vi "Start LabVIEW.vi"(8 "Error In":errorcluster, 11 "Install LV Data":T1={"SSH Session"=refnum, "Status Log"="", "Detailed Log"="", "Credentials"={"Hostname or IP"="192.168.7.2", "Username"="root", "Password"=""}, "Target Info"={"OS Version"="", "CPU"="", "Systemd Version"="", "Internet Access"=FALSE, "Device Type"="", "LV Installed Ver"="", "LV Available Ver"="", "LV Upgrade Available"=FALSE, "Hostname"="", "NIC Info"=[]}, "Reboot Required?"=FALSE}) -> (0 "Error Out":errorcluster, 1 "Log":string, 2 "LV Running?":bool, 3 "Install LV Data":T1={"SSH Session"=refnum, "Status Log"="", "Detailed Log"="", "Credentials"={"Hostname or IP"="192.168.7.2", "Username"="root", "Password"=""}, "Target Info"={"OS Version"="", "CPU"="", "Systemd Version"="", "Internet Access"=FALSE, "Device Type"="", "LV Installed Ver"="", "LV Available Ver"="", "LV Upgrade Available"=FALSE, "Hostname"="", "NIC Info"=[]}, "Reboot Required?"=FALSE})   [LabVIEW 2019, in "LMH-LINX.lvlib"]
uses:
  <vilib>/MakerHub/LINX/LMH-LINX.lvlib
  <vilib>/MakerHub/LINX/Private/Utilties/Target Management/Install LV Data.ctl
  E:/lv2019/dist/vi.lib/MakerHub/LINX/Resources/Renci.SshNet.dll
  Resources/Renci.SshNet.dll
  <vilib>/MakerHub/LINX/Private/Utilties/Target Management/Target Info.ctl
  <vilib>/MakerHub/LINX/Private/Utilties/Target Management/NIC Info.ctl
  <vilib>/MakerHub/LINX/Private/Utilties/Target Management/NIC Mode.ctl
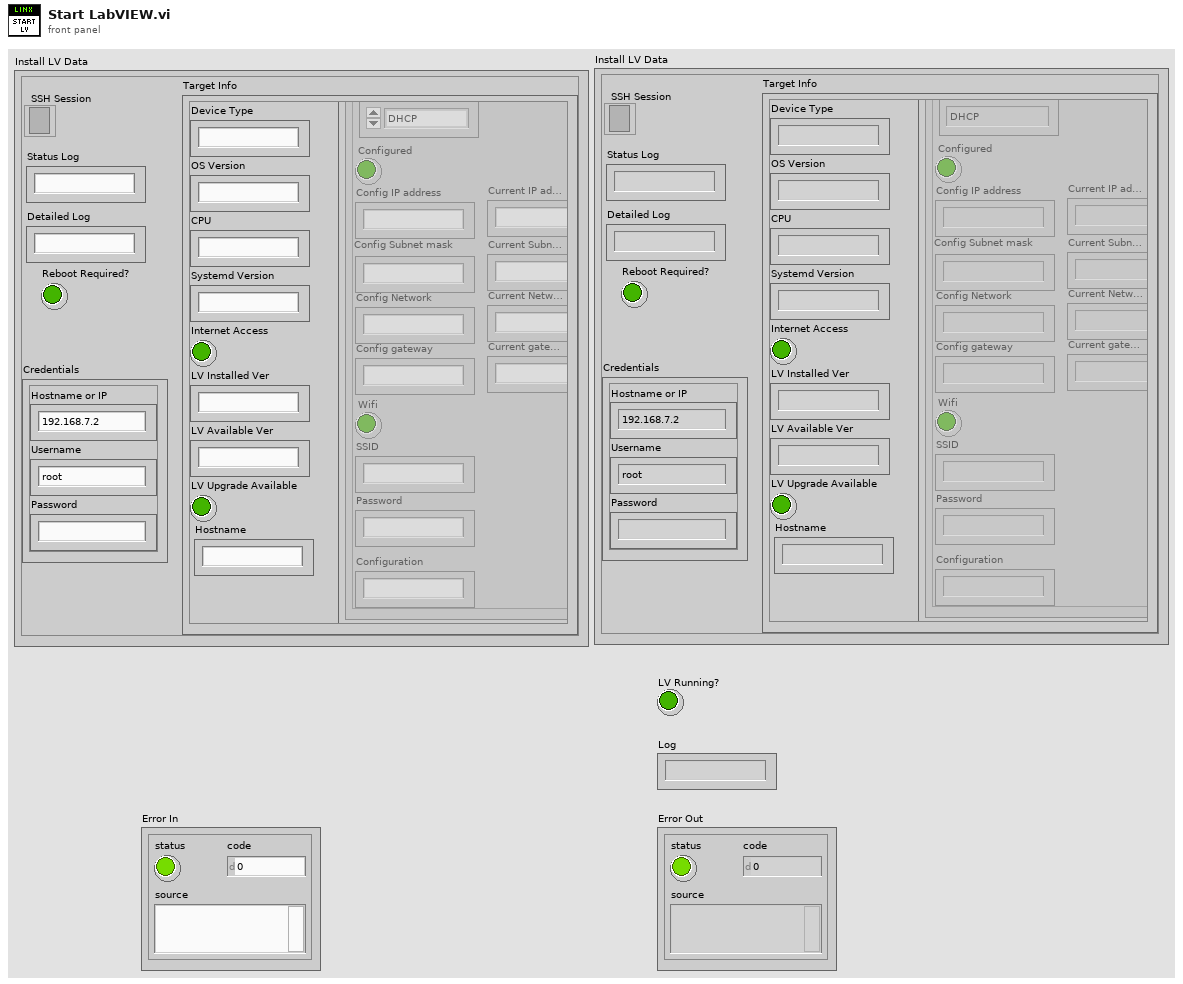
[diagram p1: front panel]
types:
  T1 = typedef "LMH-LINX.lvlib/Install LV Data.ctl" = cluster{"SSH Session":refnum<k24>, "Status Log":string, "Detailed Log":string, "Credentials":cluster{"Hostname or IP":string, "Username":string, "Password":string}, "Target Info":T2, "Reboot Required?":bool}
  T2 = typedef "LMH-LINX.lvlib/Target Info.ctl" = cluster{"OS Version":string, "CPU":string, "Systemd Version":string, "Internet Access":bool, "Device Type":string, "LV Installed Ver":string, "LV Available Ver":string, "LV Upgrade Available":bool, "Hostname":string, "NIC Info":T3[]}
  T3 = typedef "LMH-LINX.lvlib/NIC Info.ctl" = cluster{"Name":string, "NIC Mode":T4, "Configured":bool, "Config IP address":string, "Config Subnet mask":string, "Config Network":string, "Config gateway":string, "Wifi":bool, "SSID":string, "Password":string, "Configuration":string, "Current IP address":string, "Current Subnet mask":string, "Current gateway":string, "Current Network":string}
  T4 = typedef "LMH-LINX.lvlib/NIC Mode.ctl" = enum16{"DHCP", "Static", "Loopback"}
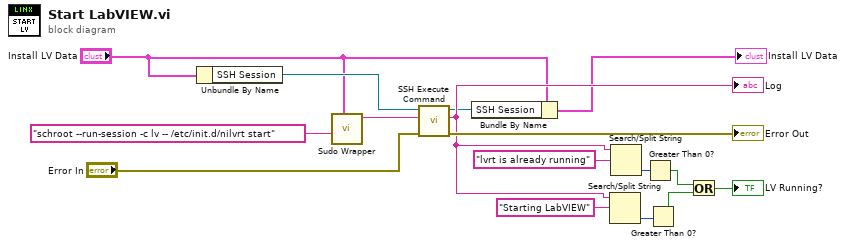
[diagram p0: block diagram]
diagram:
  n1 = Unbundle By Name("Install LV Data") -> ("SSH Session"=w6:refnum<k24>)
  n2 = call <vilib>:"Sudo Wrapper.vi"("Install LV Data"="Install LV Data", "comand string"="schroot --run-session -c lv -- /etc/init.d/nilvrt start") -> ("combined command string"=w2:string)  [unwired: 9 in]
  n3 = call <vilib>:"SSH Execute Command.vi"("Error In"="Error In", "Command"=w2, "SSH Session"=w6) -> ("Error Out"=→"Error Out":errorcluster, "Std Out"=w8:string, "SSH Session"=w5:refnum<k24>)  [unwired: 6 in]
  "Log" <- w8
  n4 = Bundle By Name(cluster="Install LV Data", "SSH Session"=w5) -> (→"Install LV Data":T1)
  n5 = Search/Split String(string=w8, search string/char (-)="Starting LabVIEW" ("regular expression")) -> (offset of match=w10:i32)  [unwired: 1 in, 2 out]
  n6 = Search/Split String(string=w8, search string/char (-)="lvrt is already running" ("regular expression")) -> (offset of match=w12:i32)  [unwired: 1 in, 2 out]
  n7 = Greater Than 0?(x=w12) -> (x > 0?=w11:bool)
  n8 = Greater Than 0?(x=w10) -> (x > 0?=w9:bool)
  n9 = Or(x=w11, y=w9) -> (x .or. y?=→"LV Running?":bool)
